vi "Test_WriteValue_CheckStrings_StringsUpdated.vi"(8 "error in (no error)":errorcluster, 11 "TestCase in":refnum<class "TestRingStringsBinding.lvclass">) -> (0 "error out":errorcluster, 3 "TestCase out":refnum<class "TestRingStringsBinding.lvclass">)   [LabVIEW 2017, in "TestRingStringsBinding.lvclass"]
uses:
  TestRingStringsBinding.lvclass
  Source/Concrete/RingStringsBinding/RingStringsBinding.lvclass
  C:/Git/composed-transport/Source/ITransport/ITransport.lvclass
  Source/ITransport/ITransport.lvclass
panel:
  in  "Ring":u16(ring) items=["a", "b", "c"]
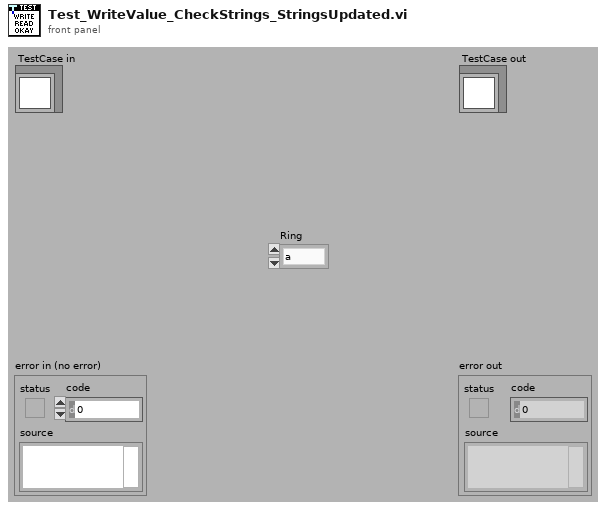
[diagram p1: front panel]
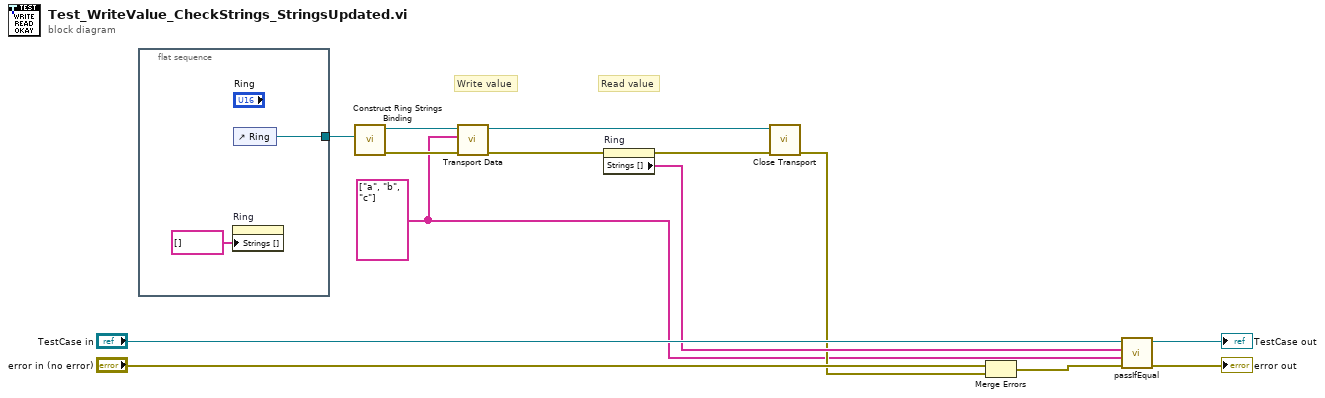
[diagram p0: block diagram]
diagram:
  w1 = string[] ["a", "b", "c"]
  # "Read value"
  # "Write value"
  n1 = flat-sequence {
    tunnel: [w16] -> w6
    frame #0 {
      n2 = property on="Ring" class="Ring (strict)"("Strings []"=string[] []) -> ()  [unwired: 2 in, 2 out]
      n3 = control-ref of="Ring"() -> (w16:refnum<vi>)
    }
  }
  n4 = call "Construct Ring Strings Binding.vi"("Ring Refnum"=w6) -> ("error out"=w8:errorcluster, "RingStringsBinding"=w10:refnum<class "RingStringsBinding.lvclass">)  [unwired: 9 in]
  n5 = call "Transport Data.vi"("error in (no error)"=w8, "Value"=w1, "ITransport in"=w10) -> ("error out"=w5:errorcluster, "ITransport out"=w7:refnum<class "RingStringsBinding.lvclass">)  [unwired: 7 in]
  n6 = property on="Ring" class="Ring (strict)"(error in=w5) -> (error out=w4:errorcluster, "Strings []"=w3:string[])  [unwired: 1 in, 1 out]
  n7 = call-dynamic "Close Transport.vi"("error in (no error)"=w4, "ITransport in"=w7) -> ("error out"=w2:errorcluster)  [unwired: 9 in]
  n8 = Merge Errors("error in (no error)", w2) -> (w9:errorcluster)
  n9 = call-dynamic "passIfEqual.vi"("error in (no error)"=w9, "y"=w1, "x"=w3, "TestCase in"="TestCase in") -> ("error out"=→"error out":errorcluster, "TestCase out"=→"TestCase out":refnum<class "TestRingStringsBinding.lvclass">)  [unwired: 6 in]
